vi "test_get_testimages.vi"() -> ()   [LabVIEW 2018, in "LV2Julia_examples.lvlib"]
uses:
  LV2Julia_examples.lvlib
  LV2Julia_core/VIs/Server or client state.ctl
  LV2Julia_core/VIs/detailed error info.ctl
  LV2Julia_core/VIs/StackFrame.ctl
  LV2Julia_core/VIs/Commands.ctl
  b3d2dca1-5e2b-4c2b-a3b1-37e7c47fa7d2.vi
  18e075e7-4cd2-4762-b22d-c93500a3c2e5.vi
  b3d2dca1-5e2b-4c2b-a3b1-37e7c47fa7d2.vi/efdc4f33-50a6-4b77-a441-768b666ba48d.vi
  18e075e7-4cd2-4762-b22d-c93500a3c2e5.vi/cc287e86-7f7c-4d41-b411-1247f41b8c10.vi
  b3d2dca1-5e2b-4c2b-a3b1-37e7c47fa7d2.vi/efdc4f33-50a6-4b77-a441-768b666ba48d.vi/eb534995-b14e-42f8-b455-e004d85ef123.vi
  b3d2dca1-5e2b-4c2b-a3b1-37e7c47fa7d2.vi/efdc4f33-50a6-4b77-a441-768b666ba48d.vi/01500c97-7bf3-4a20-a11b-bbc34a88fbfd.vi
  b3d2dca1-5e2b-4c2b-a3b1-37e7c47fa7d2.vi/efdc4f33-50a6-4b77-a441-768b666ba48d.vi/74dfd828-ee70-4a07-8c1a-a7607c190555.vi
  18e075e7-4cd2-4762-b22d-c93500a3c2e5.vi/cc287e86-7f7c-4d41-b411-1247f41b8c10.vi/f6feef97-0d99-4abe-9a13-f5c431160f6b.vi
  18e075e7-4cd2-4762-b22d-c93500a3c2e5.vi/cc287e86-7f7c-4d41-b411-1247f41b8c10.vi/31373838-9fd9-4c1b-bad6-713cb78900ae.vi
  18e075e7-4cd2-4762-b22d-c93500a3c2e5.vi/cc287e86-7f7c-4d41-b411-1247f41b8c10.vi/08ac2869-d124-46da-b7f1-aa2e040955cc.vi
  LV2Julia_core/VIs/check ID validity.vi
  LV2Julia_core/VIs/bindata_descr to JSON.vi
  LV2Julia_core/VIs/check cluster field names.vi
  LV2Julia_core/VIs/concat JSON.vi
  LV2Julia_core/VIs/build request.vi
  LV2Julia_core/VIs/Parse server response.vi
  LV2Julia_core/VIs/log jl exceptions.vi
  LV2Julia_core/LV2Julia_core.lvlib
panel:
  out "picture":picture
  out "detailed error info 2":T1
  in  "select image":u16(ring) items=["autumn_leaves.png", "blobs.gif", "cameraman.tif", "chelsea.png", "coffee.png", "earth_apollo17.jpg", "fabio_color_256.png", "fabio_color_512.png", "fabio_gray_256.png", "fabio_gray_512.png", "hela-cells.tif", "house.tif", "jetplane.tif", "lake_color.tif", "lake_gray.tif", "lena_color_256.tif", "lena_color_512.tif", "lena_gray_256.tif", "lena_gray_512.tif", "lena_gray_16bit.png", "livingroom.tif", "lighthouse.png", "mandril_color.tif", "mandril_gray.tif", "mandrill.tiff", "m51.tif", "moonsurface.tiff", "mountainstream.png", "peppers_color.tif", "peppers_gray.tif", "pirate.tif", "resolution_test_512.tif", "resolution_test_1920.tif", "toucan.png", "walkbridge.tif", "woman_blonde.tif", "woman_darkhair.tif"]
  in  "Start Server from LabVIEW":bool=TRUE
  in  "next":bool
  in  "stop LV only":bool
  in  "stop":bool
  out "detailed error info":T1
  out "Jl Server state out":T3
  out "final error":errorcluster
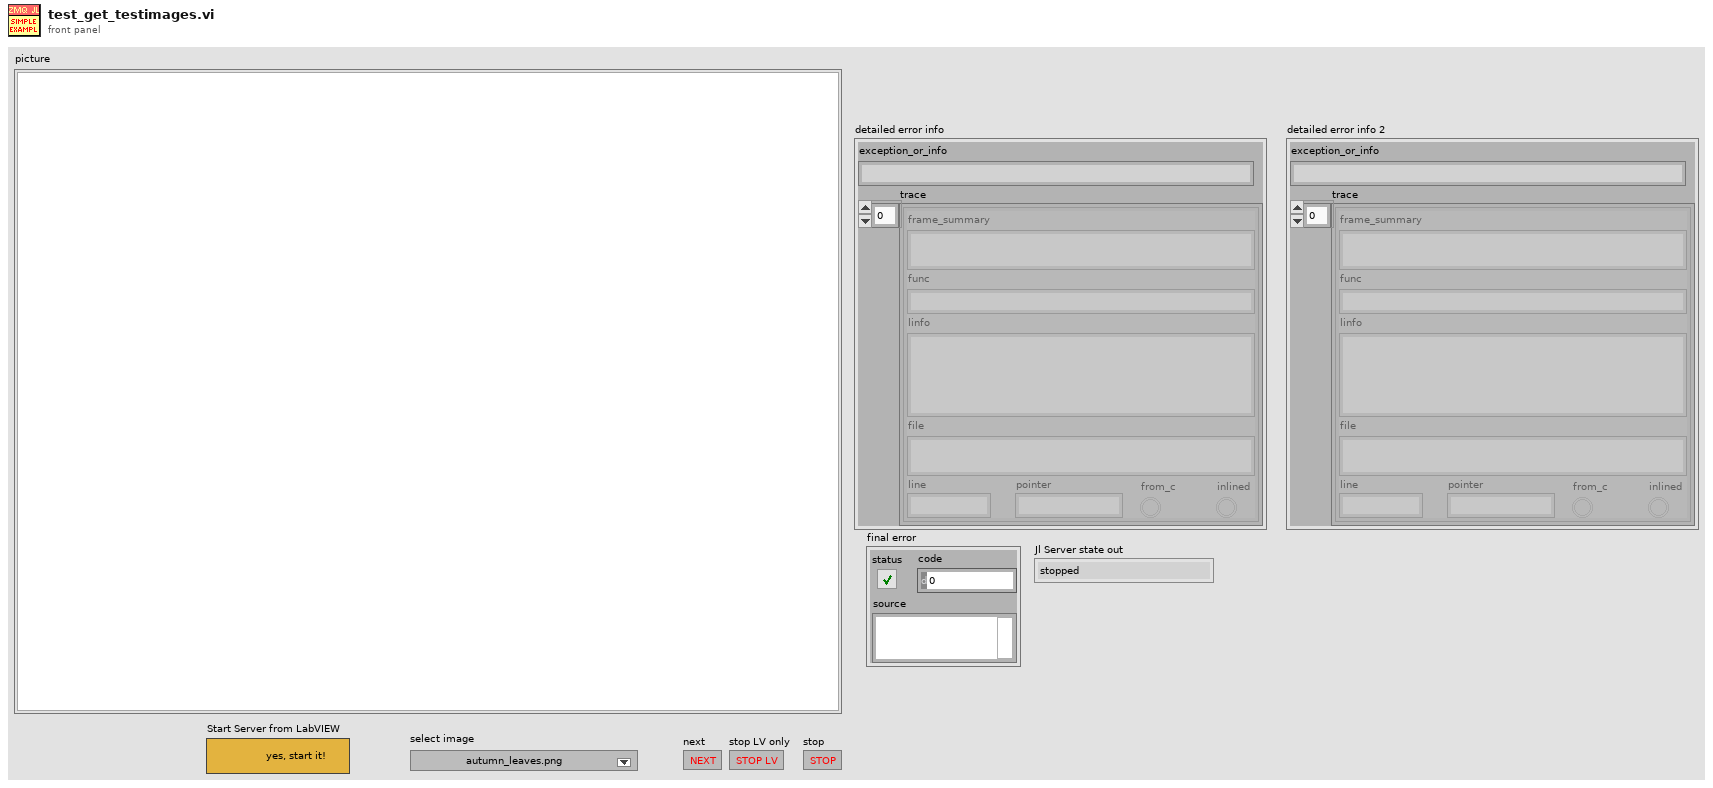
[diagram p1: front panel]
types:
  T1 = typedef "LV2Julia_core.lvlib/detailed error info.ctl" = cluster{"exception_or_info":string, "trace":T2[]}
  T2 = typedef "LV2Julia_core.lvlib/StackFrame.ctl" = cluster{"frame_summary":string, "func":string, "linfo":string, "file":string, "line":i32, "pointer":u64, "from_c":bool, "inlined":bool}
  T3 = typedef "LV2Julia_core.lvlib/Server or client state.ctl" = enum16{"stopped", "running", "unknown"}
  T4 = typedef "LV2Julia_core.lvlib/Commands.ctl" = enum16{"Start Jl-server & Init LV-client", "Send request & Get response ", "Stop Jl-server & Cleanup LV-client", "Cleanup LV-client", "Start Jl-server", "Stop Jl-server", "Init LV-Client", "Cleanup LV-Client", "(not allowed)", "Set LV Client state", "Set Jl Server state", "set ZMQ timeout", "read ZMQ timeout", "read-out state"}
  T5 = typedef "imagedata.ctl" = cluster{"image type":i32, "image depth":i32, "image":u8[], "mask":u8[], "colors":u32[], "Rectangle":cluster{"left":i16, "top":i16, "right":i16, "bottom":i16}}
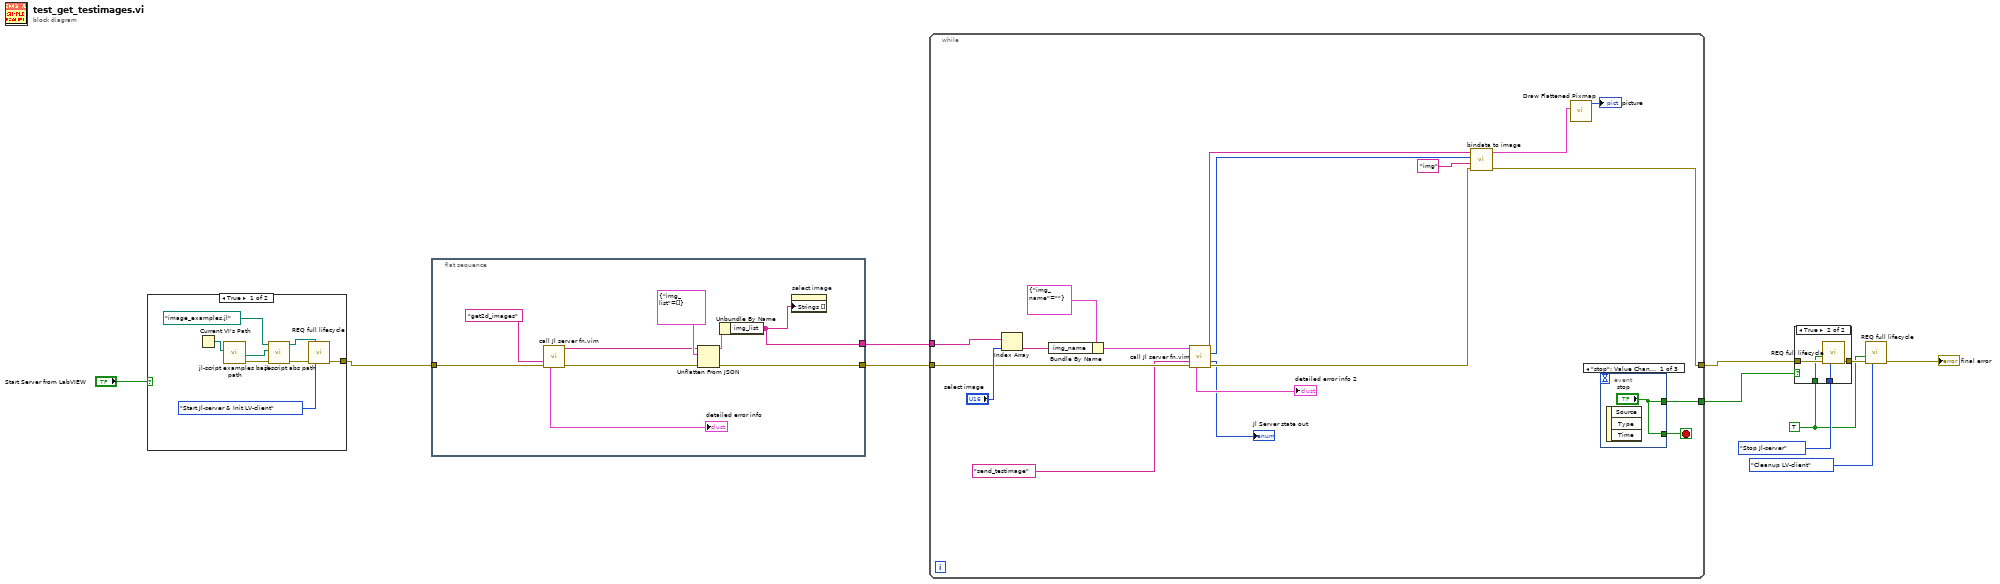
[diagram p0: block diagram]
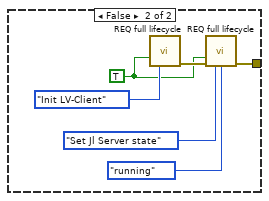
[diagram p2: hidden frame]
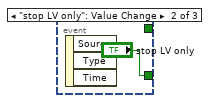
[diagram p3: hidden frame]
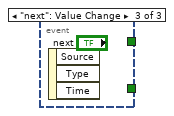
[diagram p4: hidden frame]
diagram:
  w7 = TRUE ("Force command")
  n1 = case shown="True" "Start Server from LabVIEW" {
    tunnel: [w18 w20] -> w4
    frame True {
      n2 = Current VI's Path() -> (path=w14:path)
      n3 = call "jl-script examples base path.vi"("calling example VI path"=w14) -> ("error out"=w13:errorcluster, "jl-script-examples base path"=w12:path)  [unwired: 9 in]
      n4 = call "jl-script abs path.vi"("error in (no error)"=w13, "Base path (not a path)"=w12, "Julia user functions script"=path "image_examples.jl") -> ("error out"=w15:errorcluster, "script abs path"=w16:path)  [unwired: 7 in]
      n5 = call "REQ full lifecycle.vi"("Julia user functions script"=w16, "error in"=w15, "command"=Commands."Start Jl-server & Init LV-client") -> ("error out"=w18:errorcluster)  [unwired: 6 in, 6 out]
    }
    frame False {
      w22 = TRUE ("Force command")
      n6 = call "REQ full lifecycle.vi"("Force command"=w22, "command"=Commands."Init LV-Client") -> ("error out"=w24:errorcluster)  [unwired: 7 in, 6 out]
      n7 = call "REQ full lifecycle.vi"("Force command"=w22, "error in"=w24, "command"=Commands."Set Jl Server state", "Jl Server state in"=Server_or_client_state."running") -> ("error out"=w20:errorcluster)  [unwired: 5 in, 6 out]
    }
  }
  n8 = flat-sequence {
    tunnel: [w34] -> w3
    tunnel: w4 -> [w29]
    tunnel: [w31] -> w1
    frame #0 {
      n9 = call "call Jl server fn.vim"("fun2call"="get2d_images", "error in (no error)"=w29) -> ("JSON received"=w28:string, "detailed error info"=→"detailed error info":T1, "error out"=w27:errorcluster)  [unwired: 7 in, 4 out]
      n10 = Unflatten From JSON(JSON string=w28, type and defaults=cluster{"img_list":string[]} {"img_list"=[]} ("parsed response"), error in (no error)=w27) -> (value=w32:cluster{"img_list":string[]}, error out=w34:errorcluster)  [unwired: 4 in]
      n11 = Unbundle By Name(w32) -> ("img_list"=w31:string[])
      n12 = property on="select image" class="Ring (strict)"("Strings []"=w31) -> ()  [unwired: 2 in, 2 out]
    }
  }
  n13 = while {
    tunnel: [w51] -> w6
    tunnel: w3 -> [w42]
    tunnel: [w46] -> w2
    tunnel: w1 -> [w50]
    stop <- w52 stop-if-true
    n14 = Index Array(array=w50, index="select image") -> (element=w47:string)
    n15 = Bundle By Name(cluster=cluster{"img_name":string} {"img_name"=""} ("parsed response"), "img_name"=w47) -> (w40:cluster{"img_name":string})
    n16 = call "call Jl server fn.vim"("Arguments 1"=w40, "fun2call"="send_testimage", "error in (no error)"=w42) -> ("JSON received"=w38:string, "binary data received"=w39:u8[], "Jl Server state out"=→"Jl Server state out":T3, "detailed error info"=→"detailed error info 2":T1, "error out"=w43:errorcluster)  [unwired: 6 in, 2 out]
    n17 = call "bindata to image.vi"("error in (no error)"=w43, "name"="img", "binary data in"=w39, "JSON in"=w38) -> ("error out"=w46:errorcluster, "img out"=w44:T5)  [unwired: 6 in]
    n18 = call <vilib>:"Draw Flattened Pixmap.vi"("image data"=w44) -> ("new picture"=→"picture":picture)  [unwired: 8 in]
    n19 = event shown="[0] \"stop\": Value Change" {
      selector: _ -> [_ _ _]
      dyn-events: _ -> [_ _ _]
      timeout: _ -> [_ _ _]
      tunnel: ["stop" "stop LV only" _] -> w52
      tunnel: ["stop" _ _] -> w51
      event "stop": Value Change {
        n20 = event-data() -> ()  [unwired: 1 in, 3 out]
      }
      event "stop LV only": Value Change {
        n21 = event-data() -> ()  [unwired: 1 in, 3 out]
      }
      event "next": Value Change {
        n22 = event-data() -> ()  [unwired: 1 in, 3 out]
      }
    }
  }
  n23 = case shown="True" w6 {
    tunnel: w2 -> [w55 w59]
    tunnel: Commands."Stop Jl-server" ("command") -> [_ w58]
    tunnel: [w55 w57] -> w10
    tunnel: w7 -> [_ w56]
    frame False {
    }
    frame True {
      n24 = call "REQ full lifecycle.vi"("Force command"=w56, "error in"=w59, "command"=w58) -> ("error out"=w57:errorcluster)  [unwired: 6 in, 6 out]
    }
  }
  n25 = call "REQ full lifecycle.vi"("Force command"=w7, "error in"=w10, "command"=Commands."Cleanup LV-client") -> ("error out"=→"final error":errorcluster)  [unwired: 6 in, 6 out]
